vi "StreamEngine.StartCmd.Send.vi"(8 "error in (no error)":errorcluster, 9 "Project Folder":path, 10 "gRPC Info":T1, 11 "Q Refs":T4) -> (0 "error out":errorcluster)   [LabVIEW 2025, in "XNET Bus Monitor Client.lvlib"]
uses:
  XNET Bus Monitor Client.lvlib
  Types/StreamEngine.QueueRefs.ctl
  Types/StreamEngine.CmdQueueData.ctl
  Types/StreamEngine.CmdQueueData.Cmd.ctl
  Types/SubProcessEngine.QueueRefs.ctl
  Types/SubProcessEngine.CmdQueueData.ctl
  Types/SubProcessEngine.CmdQueueData.Cmd.ctl
  Types/gRPC.ConnectionInfo.ctl
  <vilib>/gRPC/LabVIEW gRPC Library/Shared/grpcId.ctl
  bus_monitor_client/RPC Messages/ni_bus_monitor_api_Session.ctl
  Types/StreamEngine.CmdQueueData.InitialSettings.ctl
  <vilib>/gRPC/LabVIEW gRPC Library/grpc-lvsupport-release.lvlib
  bus_monitor_client/bus_monitor_client.lvlib
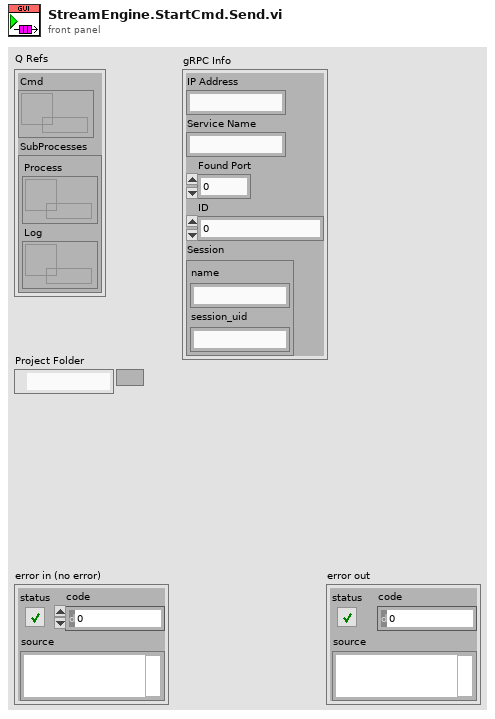
[diagram p1: front panel]
types:
  T1 = typedef "XNET Bus Monitor Client.lvlib/gRPC.ConnectionInfo.ctl" = cluster{"IP Address":string, "Service Name":string, "Found Port":u64, "ID":T2, "Session":T3}
  T2 = typedef "grpc-lvsupport-release.lvlib/grpcId.ctl" = u64
  T3 = typedef "bus_monitor_client.lvlib/ni_bus_monitor_api_Session.ctl" = cluster{"name":string, "session_uid":string}
  T4 = typedef "XNET Bus Monitor Client.lvlib/StreamEngine.QueueRefs.ctl" = cluster{"Cmd":refnum<queue>, "SubProcesses":T5}
  T5 = typedef "XNET Bus Monitor Client.lvlib/SubProcessEngine.QueueRefs.ctl" = cluster{"Process":refnum<queue>, "Log":refnum<queue>}
  T6 = typedef "XNET Bus Monitor Client.lvlib/StreamEngine.CmdQueueData.InitialSettings.ctl" = cluster{"gRPC ID":T2, "Session":T3, "Project Folder":path}
  T7 = typedef "XNET Bus Monitor Client.lvlib/StreamEngine.CmdQueueData.Cmd.ctl" = enum8{"Start Stream", "Stop Stream", "Exit"}
  T8 = typedef "XNET Bus Monitor Client.lvlib/StreamEngine.CmdQueueData.ctl" = cluster{"Cmd":T7, "Parameters":variant}
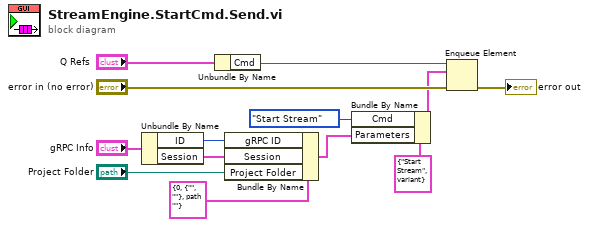
[diagram p0: block diagram]
diagram:
  n1 = Unbundle By Name("gRPC Info") -> ("ID"=w2:T2, "Session"=w1:T3)
  n2 = Unbundle By Name("Q Refs") -> ("Cmd"=w9:refnum<queue>)
  n3 = Bundle By Name(cluster=T6 {"gRPC ID"=0, "Session"={"name"="", "session_uid"=""}, "Project Folder"=path ""}, "gRPC ID"=w2, "Session"=w1, "Project Folder"="Project Folder") -> (w5:T6)
  n4 = Bundle By Name(cluster=T8 {"Cmd"=enum."Start Stream", "Parameters"=variant} ("element"), "Cmd"=StreamEngine.CmdQueueData.Cmd."Start Stream", "Parameters"=w5) -> (w10:T8)
  n5 = Enqueue Element(queue=w9, element=w10, error in (no error)="error in (no error)") -> (error out=→"error out":errorcluster)  [unwired: 1 in, 2 out]
